vi "Create Cell.vi"(0 "Leading":T2=18.0, 2 "Text rotation":T1, 5 "Font Ref":refnum<k24>, 7 "Vertical Alignement":T3, 9 "Cell Appearance":T4={"Border"=0, "Thickness"=0.5, "Color"=0, "BG"=16777225}, 11 "error in (no error)":errorcluster) -> (8 "PdfP Cell ref":refnum<k24>, 15 "error out":errorcluster)   [LabVIEW 2020, in "Exaprom PDF.lvlib"]
doc: "Version 1.0\nDeveloped by Jean-Marc Simard\nCopyright © 2010, Exaprom Inc.\nAll rights reserved.\nLicense: BSD\n\nWith iTextSharp 4.1.6 (http://itextsharp.sourceforge.net)\nunder Mozilla Public License Version 1.1\n(http://www.mozilla.org/MPL/MPL-1.1.html)"
uses:
  <userlib>/labview-PDF-writer-master/Exaprom PDF.lvlib
  C:/Program Files (x86)/National Instruments/LabVIEW 2020/user.lib/labview-PDF-writer-master/DLL/itextsharp.dll
  DLL/itextsharp.dll
  <userlib>/labview-PDF-writer-master/Controls/Table Controls/Cell Appearance.ctl
  <userlib>/labview-PDF-writer-master/Controls/Table Controls/Cell Border 20 px.ctl
  <userlib>/labview-PDF-writer-master/Controls/Table Controls/Cell Vertical alignment.ctl
  <userlib>/labview-PDF-writer-master/Controls/Font Controls/Font size.ctl
  <userlib>/labview-PDF-writer-master/Controls/Table Controls/Text vertical arrangement.ctl
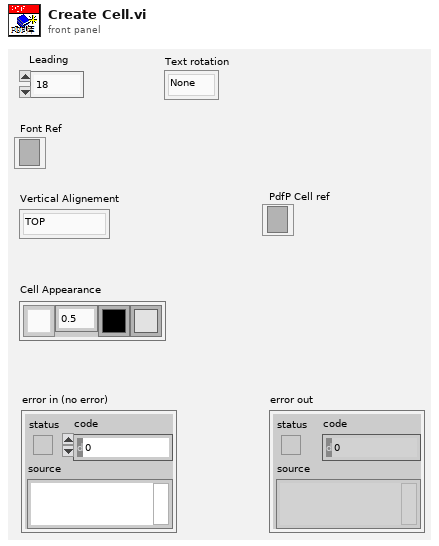
[diagram p1: front panel]
types:
  T1 = typedef "Exaprom PDF.lvlib/Text vertical arrangement.ctl" = enum16{"None", "Clockwise", "Counterclockwise"}
  T2 = typedef "Exaprom PDF.lvlib/Font size.ctl" = sgl
  T3 = typedef "Exaprom PDF.lvlib/Cell Vertical alignment.ctl" = enum16{"TOP", "MIDDLE", "BOTTOM"}
  T4 = typedef "Exaprom PDF.lvlib/Cell Appearance.ctl" = cluster{"Border":T5, "Thickness":sgl, "Color":u32, "BG":u32}
  T5 = typedef "Exaprom PDF.lvlib/Cell Border 20 px.ctl" = u16
  T6 = typedef "Exaprom PDF.lvlib/Cell Border iText number.ctl" = u16
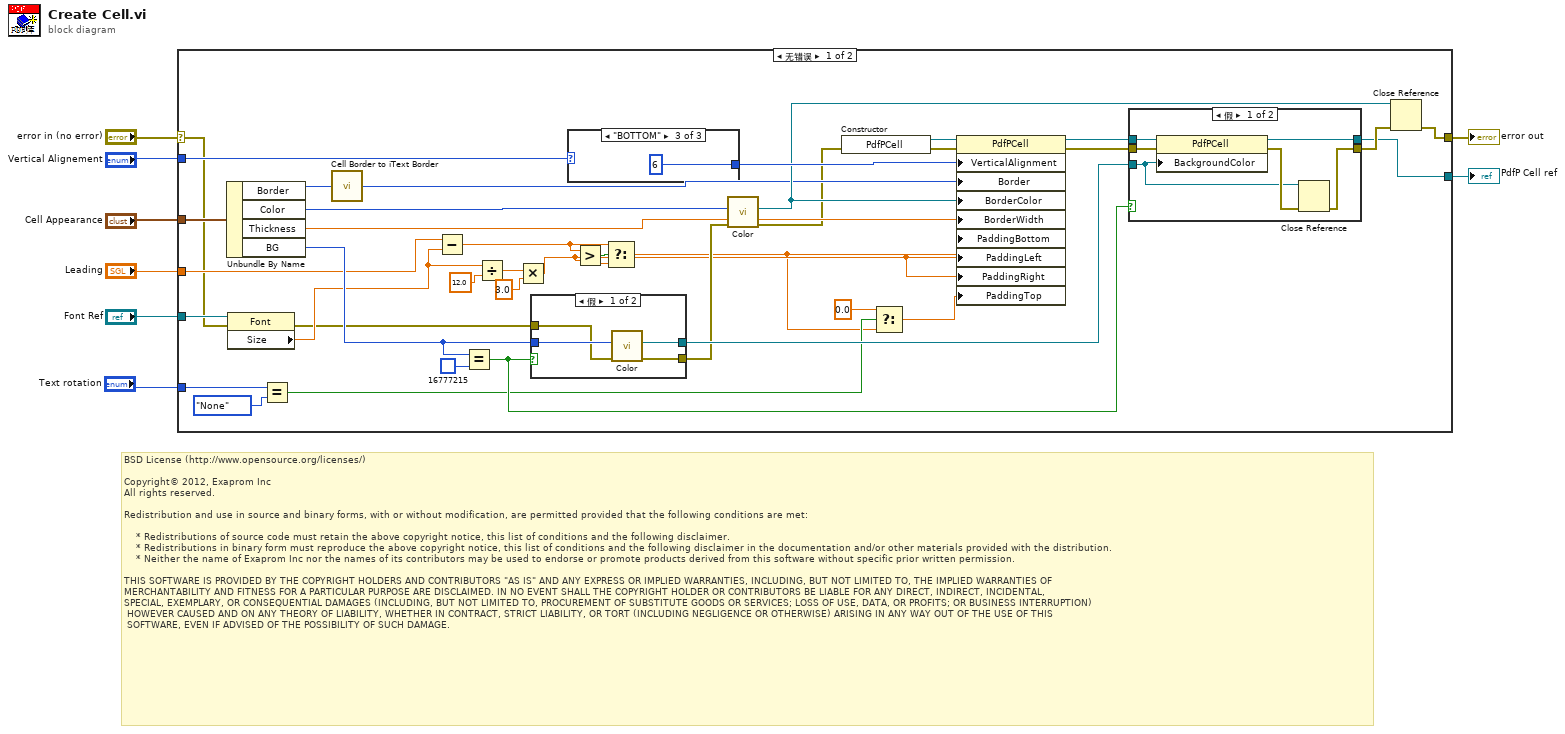
[diagram p0: block diagram]
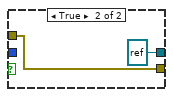
[diagram p2: hidden frame]
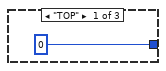
[diagram p4: hidden frame]
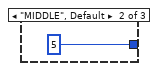
[diagram p5: hidden frame]
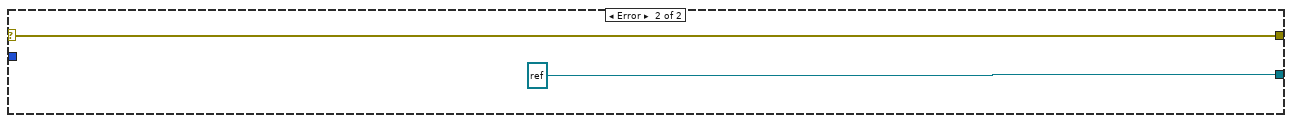
[diagram p6: hidden frame]
diagram:
  # "BSD License (http://www.opensource.org/licenses/)\n\nCopyright© 2012, Exaprom Inc\nAll rights reserved.\n\nRedistribution and use in source and binary forms, with or without modification, are permitted provided that the following conditions are met:\n\n    * Redistributions of source code must retain the above copyright notice, this list of conditions and the following disclaimer.\n    * Redistributions in binary form must reproduce the above copyright notice, this list of conditions and the following disclaimer in the documentation and/or other materials provided with the distribution.\n    * Neither the name of Exaprom Inc nor the names of its contributors may be used to endorse or promote products derived from this software without specific prior written permission.\n\nTHIS SOFTWARE IS PROVIDED BY THE COPYRIGHT HOLDERS AND CONTRIBUTORS \"AS IS\" AND ANY EXPRESS OR IMPLIED WARRANTIES, INCLUDING, BUT NOT LIMITED TO, THE IMPLIED WARRANTIES OF \nMERCHANTABILITY AND FITNESS FOR A PARTICULAR PURPOSE ARE DISCLAIMED. IN NO EVENT SHALL THE COPYRIGHT HOLDER OR CONTRIBUTORS BE LIABLE FOR ANY DIRECT, INDIRECT, INCIDENTAL,\nSPECIAL, EXEMPLARY, OR CONSEQUENTIAL DAMAGES (INCLUDING, BUT NOT LIMITED TO, PROCUREMENT OF SUBSTITUTE GOODS OR SERVICES; LOSS OF USE, DATA, OR PROFITS; OR BUSINESS INTERRUPTION)\n HOWEVER CAUSED AND ON ANY THEORY OF LIABILITY, WHETHER IN CONTRACT, STRICT LIABILITY, OR TORT (INCLUDING NEGLIGENCE OR OTHERWISE) ARISING IN ANY WAY OUT OF THE USE OF THIS\n SOFTWARE, EVEN IF ADVISED OF THE POSSIBILITY OF SUCH DAMAGE."
  n1 = case shown="无错误" "error in (no error)" {
    selector: "error in (no error)" -> [w16 w65]
    tunnel: [w34 w65] -> w7
    tunnel: [w35 refnum<k24> refnum ("new reference")] -> w6
    tunnel: "Cell Appearance" -> [w43 _]
    tunnel: "Vertical Alignement" -> [w28 _]
    tunnel: "Leading" -> [w22 _]
    tunnel: "Font Ref" -> [w21 _]
    tunnel: "Text rotation" -> [w15 _]
    frame No Error {
      n2 = Unbundle By Name(w43) -> ("Border"=w27:T5, "Color"=w25:u32, "Thickness"=w24:sgl, "BG"=w23:u32)
      n3 = property class="Font"(reference=w21, error in=w16) -> (error out=w17:errorcluster, "Size"=w18:sgl)  [unwired: 1 out]
      n4 = Equal?(x=w15, y=Text_vertical_arrangement."None" ("Text rotation")) -> (x = y?=w12:bool)
      n5 = call <userlib>:"Cell Border to iText Border.vi"("Cell Border"=w27) -> ("Cell Border iText value"=w26:T6)  [unwired: 14 in]
      n6 = Subtract(x=w22, y=w18) -> (x-y=w44:T2)
      n7 = Equal?(x=w23, y=u32 16777215 ("Color")) -> (x = y?=w32:bool)
      n8 = Divide(x=w18, y=sgl 12.0) -> (x/y=w30:sgl)
      n9 = Multiply(x=w30, y=sgl 3.0 ("t")) -> (x*y=w11:sgl)
      n10 = case shown="假" w32 {
        tunnel: [w50 refnum<k24> refnum ("Color")] -> w37
        tunnel: w23 -> [w49 _]
        tunnel: w17 -> [w48 w51]
        tunnel: [w47 w51] -> w33
        frame False {
          n11 = call <userlib>:"Color.vi"("error in (no error)"=w48, "Color"=w49) -> ("error out"=w47:errorcluster, "Color"=w50:refnum<k24>)  [unwired: 8 out]
        }
        frame True {
        }
      }
      n12 = case shown="\"BOTTOM\"" w28 {
        tunnel: [0 5 6] -> w46
        frame "TOP" {
        }
        frame "MIDDLE", Default {
        }
        frame "BOTTOM" {
        }
      }
      n13 = Greater?(x=w44, y=w11) -> (0:w45:bool)
      n14 = Select(t=w44, s=w45, f=w11) -> (s? t:f=w9:T2)
      n15 = call <userlib>:"Color.vi"("error in (no error)"=w33, "Color"=w25) -> ("error out"=w19:errorcluster, "Color"=w38:refnum<k24>)  [unwired: 8 out]
      n16 = constructor class="PdfPCell"(error in=w19) -> (reference out=w36:refnum<k24>, error out=w20:errorcluster)  [unwired: 2 in, 1 out]
      n17 = Select(t=sgl 0.0, s=w12, f=w9) -> (s? t:f=w13:T2)
      n18 = property class="PdfPCell"(reference=w36, error in=w20, "VerticalAlignment"=w46, "Border"=w26, "BorderColor"=w38, "BorderWidth"=w24, "PaddingBottom"=w9, "PaddingLeft"=w11, "PaddingRight"=w11, "PaddingTop"=w13) -> (reference out=w39:refnum<k24>, error out=w42:errorcluster)
      n19 = case shown="假" w32 {
        tunnel: w39 -> [w58 w60]
        tunnel: w42 -> [w57 w59]
        tunnel: [w56 w60] -> w35
        tunnel: [w55 w59] -> w41
        tunnel: w37 -> [w53 _]
        frame False {
          n20 = property class="PdfPCell"(reference=w58, error in=w57, "BackgroundColor"=w53) -> (reference out=w56:refnum<k24>, error out=w54:errorcluster)
          n21 = Close Reference(reference=w53, error in (no error)=w54) -> (error out=w55:errorcluster)
        }
        frame True {
        }
      }
      n22 = Close Reference(reference=w38, error in (no error)=w41) -> (error out=w34:errorcluster)
    }
    frame Error {
    }
  }
  "error out" <- w7
  "PdfP Cell ref" <- w6
